vi "I(V)_K6221-K2182a_PK.vi"() -> ()   [LabVIEW 2016]
uses:
  Labview Drivers/Keithley 622x LV 2009/Keithley 622x.lvlib
panel:
  in  "Numeric Average":i32=50
  in  "wait (ms)":u32=1000
  out "Iset (A)":dbl=-4.3999999999999985e-06
  out "Vmeas (V)":dbl=-1.0767123e-06
  in  "Folder":path=path "D:/Banabir/Second round/14-04-2021"
  in  "Set Compliance voltage (V)":dbl=2.0 min=0.0 step=0.1 format="%_3f"
  out "I vs V":cluster{dbl, "Field Reading":dbl}[](graph)=[{-2.65213861e-07, "Field Reading"=0.0}, {-2.06331562e-07, "Field Reading"=1e-07}, {-2.45753416e-07, "Field Reading"=2e-07}, {-2.41658661e-07, "Field Reading"=3e-07}, {-2.45242211e-07, "Field Reading"=4e-07}, {-2.44727893e-07, "Field Reading"=5e-07}, {-1.955806e-07, "Field Reading"=6e-07}, {-2.17089385e-07, "Field Reading"=7e-07}, {-2.81598074e-07, "Field Reading"=8e-07}, {-2.74937155e-07, "Field Reading"=9e-07}, {-2.57527922e-07, "Field Reading"=1e-06}, {-1.97112335e-07, "Field Reading"=1.1e-06}, {-1.8175889e-07, "Field Reading"=1.2e-06}, {-2.14527365e-07, "Field Reading"=1.2999999999999998e-06}, {-1.61276589e-07, "Field Reading"=1.3999999999999997e-06}, {-5.88852258e-08, "Field Reading"=1.4999999999999996e-06}, {4.14620688e-08, "Field Reading"=1.5999999999999995e-06}, {4.55608442e-08, "Field Reading"=1.6999999999999994e-06}, {1.10074806e-07, "Field Reading"=1.7999999999999993e-06}, {9.16432587e-08, "Field Reading"=1.8999999999999992e-06}, {2.22710882e-07, "Field Reading"=1.999999999999999e-06}, {2.90806804e-07, "Field Reading"=2.099999999999999e-06}, {2.74933923e-07, "Field Reading"=2.199999999999999e-06}, {2.81079697e-07, "Field Reading"=2.2999999999999987e-06}, {3.16914884e-07, "Field Reading"=2.3999999999999986e-06}, {2.95409204e-07, "Field Reading"=2.4999999999999985e-06}, {3.58898183e-07, "Field Reading"=2.5999999999999984e-06}, {3.56848457e-07, "Field Reading"=2.6999999999999983e-06}, {4.40815949e-07, "Field Reading"=2.799999999999998e-06}, {4.45430022e-07, "Field Reading"=2.899999999999998e-06}, {4.50042171e-07, "Field Reading"=2.999999999999998e-06}, {5.23763566e-07, "Field Reading"=3.099999999999998e-06}, {5.54477469e-07, "Field Reading"=3.1999999999999977e-06}, {5.89806137e-07, "Field Reading"=3.2999999999999976e-06}, {6.03627656e-07, "Field Reading"=3.3999999999999975e-06}, {6.54317135e-07, "Field Reading"=3.4999999999999974e-06}, {7.12174301e-07, "Field Reading"=3.5999999999999973e-06}, {7.36747564e-07, "Field Reading"=3.699999999999997e-06}, {8.03819501e-07, "Field Reading"=3.799999999999997e-06}, {8.68836656e-07, "Field Reading"=3.899999999999997e-06}, {9.59970204e-07, "Field Reading"=3.999999999999997e-06}, {9.96323249e-07, "Field Reading"=4.099999999999997e-06}, {1.07823925e-06, "Field Reading"=4.199999999999997e-06}, {1.11458965e-06, "Field Reading"=4.299999999999997e-06}, {1.11817613e-06, "Field Reading"=4.399999999999997e-06}, {1.23695717e-06, "Field Reading"=4.499999999999997e-06}, {1.24360737e-06, "Field Reading"=4.599999999999997e-06}, {1.27996158e-06, "Field Reading"=4.6999999999999965e-06}, {1.30914358e-06, "Field Reading"=4.799999999999996e-06}, {1.29941092e-06, "Field Reading"=4.899999999999996e-06}, {1.45659309e-06, "Field Reading"=4.999999999999996e-06}, {1.47759059e-06, "Field Reading"=5.099999999999996e-06}, {1.56462638e-06, "Field Reading"=5.199999999999996e-06}, {1.56923247e-06, "Field Reading"=5.299999999999996e-06}, {1.5958572e-06, "Field Reading"=5.399999999999996e-06}, {1.62196573e-06, "Field Reading"=5.499999999999996e-06}, {1.65985372e-06, "Field Reading"=5.5999999999999955e-06}, {1.66548618e-06, "Field Reading"=5.699999999999995e-06}, {1.73869841e-06, "Field Reading"=5.799999999999995e-06}, {1.75918207e-06, "Field Reading"=5.899999999999995e-06}, {1.82420779e-06, "Field Reading"=5.999999999999995e-06}, {1.87539735e-06, "Field Reading"=6.099999999999995e-06}, {2.02541342e-06, "Field Reading"=6.199999999999995e-06}, {2.05920615e-06, "Field Reading"=6.299999999999995e-06}, {2.0607414e-06, "Field Reading"=6.399999999999995e-06}, {2.09299708e-06, "Field Reading"=6.4999999999999945e-06}, {2.14470835e-06, "Field Reading"=6.599999999999994e-06}, {2.22560209e-06, "Field Reading"=6.699999999999994e-06}, {2.29164603e-06, "Field Reading"=6.799999999999994e-06}, {2.29522927e-06, "Field Reading"=6.899999999999994e-06}, {2.34898799e-06, "Field Reading"=6.999999999999994e-06}, {2.35974308e-06, "Field Reading"=7.099999999999994e-06}, {2.33516555e-06, "Field Reading"=7.199999999999994e-06}, {2.38277613e-06, "Field Reading"=7.299999999999994e-06}, {2.52971809e-06, "Field Reading"=7.3999999999999935e-06}, {2.52562488e-06, "Field Reading"=7.499999999999993e-06}, {2.53073687e-06, "Field Reading"=7.599999999999993e-06}, {2.67562896e-06, "Field Reading"=7.699999999999994e-06}, {2.75038341e-06, "Field Reading"=7.799999999999995e-06}, {2.77444721e-06, "Field Reading"=7.899999999999996e-06}, {2.86045666e-06, "Field Reading"=7.999999999999996e-06}, {2.95312204e-06, "Field Reading"=8.099999999999997e-06}, {2.99612267e-06, "Field Reading"=8.199999999999998e-06}, {2.98793425e-06, "Field Reading"=8.299999999999998e-06}, {3.08214364e-06, "Field Reading"=8.4e-06}, {3.07036496e-06, "Field Reading"=8.5e-06}, {3.17481336e-06, "Field Reading"=8.6e-06}, {3.13692748e-06, "Field Reading"=8.700000000000001e-06}, {3.13795104e-06, "Field Reading"=8.800000000000002e-06}, {3.21679593e-06, "Field Reading"=8.900000000000003e-06}, {3.24444364e-06, "Field Reading"=9.000000000000004e-06}, {3.34223395e-06, "Field Reading"=9.100000000000004e-06}, {3.37244308e-06, "Field Reading"=9.200000000000005e-06}, {3.49890549e-06, "Field Reading"=9.300000000000006e-06}, {3.5705844e-06, "Field Reading"=9.400000000000007e-06}, {3.56136e-06, "Field Reading"=9.500000000000007e-06}, {3.64941777e-06, "Field Reading"=9.600000000000008e-06}, {3.65403077e-06, "Field Reading"=9.700000000000009e-06}, {3.70881304e-06, "Field Reading"=9.80000000000001e-06}, {3.74413912e-06, "Field Reading"=9.90000000000001e-06}, {3.78202672e-06, "Field Reading"=1.0000000000000011e-05}, {3.77588359e-06, "Field Reading"=1.0100000000000012e-05}, {3.79482737e-06, "Field Reading"=1.0200000000000012e-05}, {3.84807257e-06, "Field Reading"=1.0300000000000013e-05}, {3.96326851e-06, "Field Reading"=1.0400000000000014e-05}, {4.02675375e-06, "Field Reading"=1.0500000000000015e-05}, {4.01548692e-06, "Field Reading"=1.0600000000000015e-05}, {4.03188336e-06, "Field Reading"=1.0700000000000016e-05}, {4.11892625e-06, "Field Reading"=1.0800000000000017e-05}, {4.16499723e-06, "Field Reading"=1.0900000000000018e-05}, {4.13786622e-06, "Field Reading"=1.1000000000000018e-05}, {4.15936464e-06, "Field Reading"=1.1100000000000019e-05}, {4.15372248e-06, "Field Reading"=1.120000000000002e-05}, {4.1921208e-06, "Field Reading"=1.130000000000002e-05}, {4.20441259e-06, "Field Reading"=1.1400000000000021e-05}, {4.22285166e-06, "Field Reading"=1.1500000000000022e-05}, {4.41023425e-06, "Field Reading"=1.1600000000000023e-05}, {4.43121181e-06, "Field Reading"=1.1700000000000024e-05}, {4.48548487e-06, "Field Reading"=1.1800000000000024e-05}, {4.51827063e-06, "Field Reading"=1.1900000000000025e-05}, {4.56332253e-06, "Field Reading"=1.2000000000000026e-05}, {4.56996768e-06, "Field Reading"=1.2100000000000026e-05}, {4.61196138e-06, "Field Reading"=1.2200000000000027e-05}, {4.66060156e-06, "Field Reading"=1.2300000000000028e-05}, {4.71282017e-06, "Field Reading"=1.2400000000000029e-05}, {4.72562207e-06, "Field Reading"=1.250000000000003e-05}, {4.80549203e-06, "Field Reading"=1.260000000000003e-05}, {4.84132842e-06, "Field Reading"=1.2700000000000031e-05}, {4.81931379e-06, "Field Reading"=1.2800000000000032e-05}, {4.91812376e-06, "Field Reading"=1.2900000000000032e-05}, {4.97443564e-06, "Field Reading"=1.3000000000000033e-05}, {5.06864178e-06, "Field Reading"=1.3100000000000034e-05}, {5.15414621e-06, "Field Reading"=1.3200000000000035e-05}, {5.14594912e-06, "Field Reading"=1.3300000000000035e-05}, {5.15516684e-06, "Field Reading"=1.3400000000000036e-05}, {5.24221524e-06, "Field Reading"=1.3500000000000037e-05}, {5.29853469e-06, "Field Reading"=1.3600000000000038e-05}, {5.35638168e-06, "Field Reading"=1.3700000000000038e-05}, {5.37020179e-06, "Field Reading"=1.3800000000000039e-05}, {5.3492118e-06, "Field Reading"=1.390000000000004e-05}, {5.39375972e-06, "Field Reading"=1.400000000000004e-05}, {5.47056068e-06, "Field Reading"=1.4100000000000041e-05}, {5.50895206e-06, "Field Reading"=1.4200000000000042e-05}, {5.5514459e-06, "Field Reading"=1.4300000000000043e-05}, {5.55707986e-06, "Field Reading"=1.4400000000000043e-05}, {5.60366331e-06, "Field Reading"=1.4500000000000044e-05}, {5.64206701e-06, "Field Reading"=1.4600000000000045e-05}, {5.75061982e-06, "Field Reading"=1.4700000000000046e-05}, {5.78440485e-06, "Field Reading"=1.4800000000000046e-05}, {5.84225116e-06, "Field Reading"=1.4900000000000047e-05}, {5.85863506e-06, "Field Reading"=1.5000000000000048e-05}, {5.91290279e-06, "Field Reading"=1.5100000000000049e-05}, {5.90009794e-06, "Field Reading"=1.520000000000005e-05}, {5.99225908e-06, "Field Reading"=1.530000000000005e-05}, {6.0357811e-06, "Field Reading"=1.540000000000005e-05}, {6.09005686e-06, "Field Reading"=1.5500000000000048e-05}, {6.16276569e-06, "Field Reading"=1.5600000000000047e-05}, {6.223172e-06, "Field Reading"=1.5700000000000046e-05}, {6.27077906e-06, "Field Reading"=1.5800000000000045e-05}, {6.31429835e-06, "Field Reading"=1.5900000000000044e-05}, {6.34911719e-06, "Field Reading"=1.6000000000000043e-05}, {6.38342782e-06, "Field Reading"=1.6100000000000042e-05}, {6.40851838e-06, "Field Reading"=1.620000000000004e-05}, {6.46738862e-06, "Field Reading"=1.630000000000004e-05}, {6.49911838e-06, "Field Reading"=1.640000000000004e-05}, {6.55799613e-06, "Field Reading"=1.650000000000004e-05}, {6.62046237e-06, "Field Reading"=1.6600000000000038e-05}, {6.63786331e-06, "Field Reading"=1.6700000000000037e-05}, {6.73360462e-06, "Field Reading"=1.6800000000000036e-05}, {6.76740248e-06, "Field Reading"=1.6900000000000035e-05}, {6.79761286e-06, "Field Reading"=1.7000000000000034e-05}, {6.87696878e-06, "Field Reading"=1.7100000000000033e-05}, {6.92663472e-06, "Field Reading"=1.7200000000000032e-05}, {6.96504415e-06, "Field Reading"=1.730000000000003e-05}, {7.05310834e-06, "Field Reading"=1.740000000000003e-05}, {7.1360323e-06, "Field Reading"=1.750000000000003e-05}, {7.18210114e-06, "Field Reading"=1.7600000000000028e-05}, {7.20208147e-06, "Field Reading"=1.7700000000000027e-05}, {7.28861423e-06, "Field Reading"=1.7800000000000026e-05}, {7.33519871e-06, "Field Reading"=1.7900000000000025e-05}, {7.44937016e-06, "Field Reading"=1.8000000000000024e-05}, {7.48215567e-06, "Field Reading"=1.8100000000000023e-05}, {7.55229248e-06, "Field Reading"=1.8200000000000022e-05}, {7.5732755e-06, "Field Reading"=1.830000000000002e-05}, {7.68847322e-06, "Field Reading"=1.840000000000002e-05}, {7.65775525e-06, "Field Reading"=1.850000000000002e-05}, {7.67208615e-06, "Field Reading"=1.860000000000002e-05}, {7.7637263e-06, "Field Reading"=1.8700000000000017e-05}, {7.84923772e-06, "Field Reading"=1.8800000000000017e-05}, {7.85384559e-06, "Field Reading"=1.8900000000000016e-05}, {7.90913653e-06, "Field Reading"=1.9000000000000015e-05}, {7.93422015e-06, "Field Reading"=1.9100000000000014e-05}, {8.02791857e-06, "Field Reading"=1.9200000000000013e-05}, {8.06375894e-06, "Field Reading"=1.9300000000000012e-05}, {8.08936091e-06, "Field Reading"=1.940000000000001e-05}, {8.13646665e-06, "Field Reading"=1.950000000000001e-05}, {8.17230556e-06, "Field Reading"=1.960000000000001e-05}, {8.25165814e-06, "Field Reading"=1.9700000000000008e-05}, {8.28083444e-06, "Field Reading"=1.9800000000000007e-05}, {8.32742883e-06, "Field Reading"=1.9900000000000006e-05}, {8.40371126e-06, "Field Reading"=2e-05}, {8.32588703e-06, "Field Reading"=1.9900000000000003e-05}, {8.27059152e-06, "Field Reading"=1.9800000000000004e-05}, {8.24550498e-06, "Field Reading"=1.9700000000000005e-05}, {8.18766651e-06, "Field Reading"=1.9600000000000005e-05}, {8.16002117e-06, "Field Reading"=1.9500000000000006e-05}, {8.11034423e-06, "Field Reading"=1.9400000000000007e-05}, {8.06631431e-06, "Field Reading"=1.930000000000001e-05}, {7.96853626e-06, "Field Reading"=1.920000000000001e-05}, {7.96494837e-06, "Field Reading"=1.910000000000001e-05}, {7.88456389e-06, "Field Reading"=1.900000000000001e-05}, {7.84667228e-06, "Field Reading"=1.8900000000000012e-05}, {7.76577688e-06, "Field Reading"=1.8800000000000013e-05}, {7.72174608e-06, "Field Reading"=1.8700000000000014e-05}, {7.70996248e-06, "Field Reading"=1.8600000000000015e-05}, {7.64032909e-06, "Field Reading"=1.8500000000000016e-05}, {7.58196852e-06, "Field Reading"=1.8400000000000017e-05}, {7.52616124e-06, "Field Reading"=1.8300000000000018e-05}, {7.43451656e-06, "Field Reading"=1.820000000000002e-05}, {7.419165e-06, "Field Reading"=1.810000000000002e-05}, {7.41302153e-06, "Field Reading"=1.800000000000002e-05}, {7.40278217e-06, "Field Reading"=1.7900000000000022e-05}, {7.34748378e-06, "Field Reading"=1.7800000000000023e-05}, {7.26146266e-06, "Field Reading"=1.7700000000000024e-05}, {7.22614421e-06, "Field Reading"=1.7600000000000025e-05}, {7.15294258e-06, "Field Reading"=1.7500000000000026e-05}, {7.13912167e-06, "Field Reading"=1.7400000000000027e-05}, {7.05105581e-06, "Field Reading"=1.7300000000000027e-05}, {7.06896784e-06, "Field Reading"=1.720000000000003e-05}, {6.98551895e-06, "Field Reading"=1.710000000000003e-05}, {6.92254427e-06, "Field Reading"=1.700000000000003e-05}, {6.86724585e-06, "Field Reading"=1.690000000000003e-05}, {6.85240011e-06, "Field Reading"=1.6800000000000032e-05}, {6.78225464e-06, "Field Reading"=1.6700000000000033e-05}, {6.77713724e-06, "Field Reading"=1.6600000000000034e-05}, {6.69368315e-06, "Field Reading"=1.6500000000000035e-05}, {6.63224313e-06, "Field Reading"=1.6400000000000036e-05}, {6.64145914e-06, "Field Reading"=1.6300000000000037e-05}, {6.55391401e-06, "Field Reading"=1.6200000000000038e-05}, {6.54776972e-06, "Field Reading"=1.610000000000004e-05}, {6.44434302e-06, "Field Reading"=1.600000000000004e-05}, {6.37830276e-06, "Field Reading"=1.590000000000004e-05}, {6.32249712e-06, "Field Reading"=1.5800000000000042e-05}, {6.30507964e-06, "Field Reading"=1.5700000000000043e-05}, {6.27589889e-06, "Field Reading"=1.5600000000000044e-05}, {6.19193872e-06, "Field Reading"=1.5500000000000045e-05}, {6.14893632e-06, "Field Reading"=1.5400000000000046e-05}, {6.10695312e-06, "Field Reading"=1.5300000000000047e-05}, {6.07315478e-06, "Field Reading"=1.5200000000000046e-05}, {6.01376066e-06, "Field Reading"=1.5100000000000045e-05}, {6.01273927e-06, "Field Reading"=1.5000000000000044e-05}, {5.94362298e-06, "Field Reading"=1.4900000000000044e-05}, {5.89037156e-06, "Field Reading"=1.4800000000000043e-05}, {5.87757219e-06, "Field Reading"=1.4700000000000042e-05}, {5.83406487e-06, "Field Reading"=1.4600000000000041e-05}, {5.7818526e-06, "Field Reading"=1.450000000000004e-05}, {5.79054303e-06, "Field Reading"=1.440000000000004e-05}, {5.72397236e-06, "Field Reading"=1.430000000000004e-05}, {5.69632955e-06, "Field Reading"=1.4200000000000039e-05}, {5.62875043e-06, "Field Reading"=1.4100000000000038e-05}, {5.61902647e-06, "Field Reading"=1.4000000000000037e-05}, {5.53097021e-06, "Field Reading"=1.3900000000000036e-05}, {5.58626586e-06, "Field Reading"=1.3800000000000036e-05}, {5.5396681e-06, "Field Reading"=1.3700000000000035e-05}, {5.49102684e-06, "Field Reading"=1.3600000000000034e-05}, {5.46030697e-06, "Field Reading"=1.3500000000000033e-05}, {5.39784099e-06, "Field Reading"=1.3400000000000033e-05}, {5.28981952e-06, "Field Reading"=1.3300000000000032e-05}, {5.3456268e-06, "Field Reading"=1.3200000000000031e-05}, {5.23811359e-06, "Field Reading"=1.310000000000003e-05}, {5.28317073e-06, "Field Reading"=1.300000000000003e-05}, {5.23554661e-06, "Field Reading"=1.2900000000000029e-05}, {5.18742312e-06, "Field Reading"=1.2800000000000028e-05}, {5.16080263e-06, "Field Reading"=1.2700000000000027e-05}, {5.08911473e-06, "Field Reading"=1.2600000000000027e-05}, {5.02306725e-06, "Field Reading"=1.2500000000000026e-05}, {4.95087495e-06, "Field Reading"=1.2400000000000025e-05}, {4.89097002e-06, "Field Reading"=1.2300000000000025e-05}, {4.85103666e-06, "Field Reading"=1.2200000000000024e-05}, {4.81161312e-06, "Field Reading"=1.2100000000000023e-05}, {4.8223712e-06, "Field Reading"=1.2000000000000022e-05}, {4.71997748e-06, "Field Reading"=1.1900000000000022e-05}, {4.70513009e-06, "Field Reading"=1.1800000000000021e-05}, {4.61860758e-06, "Field Reading"=1.170000000000002e-05}, {4.50494221e-06, "Field Reading"=1.160000000000002e-05}, {4.50442328e-06, "Field Reading"=1.1500000000000019e-05}, {4.48907395e-06, "Field Reading"=1.1400000000000018e-05}, {4.48549552e-06, "Field Reading"=1.1300000000000017e-05}, {4.43275985e-06, "Field Reading"=1.1200000000000016e-05}, {4.37336829e-06, "Field Reading"=1.1100000000000016e-05}, {4.35544798e-06, "Field Reading"=1.1000000000000015e-05}, {4.23615778e-06, "Field Reading"=1.0900000000000014e-05}, {4.18496019e-06, "Field Reading"=1.0800000000000013e-05}, {4.13529928e-06, "Field Reading"=1.0700000000000013e-05}, {4.0963864e-06, "Field Reading"=1.0600000000000012e-05}, {4.10252432e-06, "Field Reading"=1.0500000000000011e-05}, {4.14245452e-06, "Field Reading"=1.040000000000001e-05}, {4.0723185e-06, "Field Reading"=1.030000000000001e-05}, {3.99655577e-06, "Field Reading"=1.0200000000000009e-05}, {3.91820595e-06, "Field Reading"=1.0100000000000008e-05}, {3.90693848e-06, "Field Reading"=1.0000000000000008e-05}, {3.90182893e-06, "Field Reading"=9.900000000000007e-06}, {3.89824771e-06, "Field Reading"=9.800000000000006e-06}, {3.89568225e-06, "Field Reading"=9.700000000000005e-06}, {3.82297919e-06, "Field Reading"=9.600000000000005e-06}, {3.79072008e-06, "Field Reading"=9.500000000000004e-06}, {3.75283128e-06, "Field Reading"=9.400000000000003e-06}, {3.74925146e-06, "Field Reading"=9.300000000000002e-06}, {3.69600662e-06, "Field Reading"=9.200000000000002e-06}, {3.68985764e-06, "Field Reading"=9.100000000000001e-06}, {3.53830951e-06, "Field Reading"=9e-06}, {3.48967903e-06, "Field Reading"=8.9e-06}, {3.4169754e-06, "Field Reading"=8.799999999999999e-06}, {3.35195893e-06, "Field Reading"=8.699999999999998e-06}, {3.26798993e-06, "Field Reading"=8.599999999999997e-06}, {3.32840376e-06, "Field Reading"=8.499999999999997e-06}, {3.28130617e-06, "Field Reading"=8.399999999999996e-06}, {3.22038204e-06, "Field Reading"=8.299999999999995e-06}, {3.19170899e-06, "Field Reading"=8.199999999999994e-06}, {3.14817946e-06, "Field Reading"=8.099999999999994e-06}, {3.06473437e-06, "Field Reading"=7.999999999999993e-06}, {3.0155901e-06, "Field Reading"=7.899999999999992e-06}, {2.89219787e-06, "Field Reading"=7.799999999999991e-06}, {2.84355222e-06, "Field Reading"=7.69999999999999e-06}, {2.79798017e-06, "Field Reading"=7.599999999999991e-06}, {2.73245105e-06, "Field Reading"=7.499999999999991e-06}, {2.68023355e-06, "Field Reading"=7.399999999999991e-06}, {2.76420187e-06, "Field Reading"=7.299999999999991e-06}, {2.74935814e-06, "Field Reading"=7.199999999999991e-06}, {2.68791939e-06, "Field Reading"=7.099999999999991e-06}, {2.63261821e-06, "Field Reading"=6.9999999999999914e-06}, {2.60291933e-06, "Field Reading"=6.8999999999999915e-06}, {2.51843848e-06, "Field Reading"=6.799999999999992e-06}, {2.5061508e-06, "Field Reading"=6.699999999999992e-06}, {2.33208474e-06, "Field Reading"=6.599999999999992e-06}, {2.3167298e-06, "Field Reading"=6.499999999999992e-06}, {2.30443977e-06, "Field Reading"=6.399999999999992e-06}, {2.24402212e-06, "Field Reading"=6.299999999999992e-06}, {2.26142112e-06, "Field Reading"=6.199999999999992e-06}, {2.24708744e-06, "Field Reading"=6.099999999999992e-06}, {2.18258492e-06, "Field Reading"=5.9999999999999925e-06}, {2.06226311e-06, "Field Reading"=5.899999999999993e-06}, {1.97317707e-06, "Field Reading"=5.799999999999993e-06}, {1.89791536e-06, "Field Reading"=5.699999999999993e-06}, {1.8943317e-06, "Field Reading"=5.599999999999993e-06}, {1.91123261e-06, "Field Reading"=5.499999999999993e-06}, {1.79142144e-06, "Field Reading"=5.399999999999993e-06}, {1.82674468e-06, "Field Reading"=5.299999999999993e-06}, {1.75353415e-06, "Field Reading"=5.199999999999993e-06}, {1.65932968e-06, "Field Reading"=5.0999999999999935e-06}, {1.65933232e-06, "Field Reading"=4.999999999999994e-06}, {1.54669792e-06, "Field Reading"=4.899999999999994e-06}, {1.44584143e-06, "Field Reading"=4.799999999999994e-06}, {1.52673386e-06, "Field Reading"=4.699999999999994e-06}, {1.4320141e-06, "Field Reading"=4.599999999999994e-06}, {1.40795279e-06, "Field Reading"=4.499999999999994e-06}, {1.32296227e-06, "Field Reading"=4.399999999999994e-06}, {1.08181445e-06, "Field Reading"=4.299999999999994e-06}, {1.07105849e-06, "Field Reading"=4.1999999999999945e-06}, {1.07361536e-06, "Field Reading"=4.099999999999995e-06}, {1.06030613e-06, "Field Reading"=3.999999999999995e-06}, {9.90675451e-07, "Field Reading"=3.899999999999995e-06}, {9.98353274e-07, "Field Reading"=3.799999999999995e-06}, {9.51769766e-07, "Field Reading"=3.699999999999995e-06}, {9.19007087e-07, "Field Reading"=3.599999999999995e-06}, {8.96477356e-07, "Field Reading"=3.4999999999999953e-06}, {8.37598555e-07, "Field Reading"=3.3999999999999954e-06}, {7.43906148e-07, "Field Reading"=3.2999999999999955e-06}, {7.07042824e-07, "Field Reading"=3.1999999999999956e-06}, {7.8384287e-07, "Field Reading"=3.0999999999999957e-06}, {6.97316697e-07, "Field Reading"=2.999999999999996e-06}, {6.99871857e-07, "Field Reading"=2.899999999999996e-06}, {6.61988855e-07, "Field Reading"=2.799999999999996e-06}, {6.67112949e-07, "Field Reading"=2.699999999999996e-06}, {5.21710306e-07, "Field Reading"=2.5999999999999963e-06}, {5.11980802e-07, "Field Reading"=2.4999999999999964e-06}, {5.26306067e-07, "Field Reading"=2.3999999999999965e-06}, {5.57538796e-07, "Field Reading"=2.2999999999999966e-06}, {5.49862592e-07, "Field Reading"=2.1999999999999967e-06}, {4.38246539e-07, "Field Reading"=2.099999999999997e-06}, {4.53099149e-07, "Field Reading"=1.999999999999997e-06}, {3.79374306e-07, "Field Reading"=1.899999999999997e-06}, {3.25102595e-07, "Field Reading"=1.7999999999999972e-06}, {2.04792301e-07, "Field Reading"=1.6999999999999973e-06}, {2.36019239e-07, "Field Reading"=1.5999999999999974e-06}, {2.33452923e-07, "Field Reading"=1.4999999999999975e-06}, {2.2372704e-07, "Field Reading"=1.3999999999999976e-06}, {2.67761542e-07, "Field Reading"=1.2999999999999977e-06}, {2.54450874e-07, "Field Reading"=1.1999999999999978e-06}, {1.63316468e-07, "Field Reading"=1.099999999999998e-06}, {7.72994096e-08, "Field Reading"=9.99999999999998e-07}, {8.85529671e-08, "Field Reading"=8.999999999999981e-07}, {7.06354729e-08, "Field Reading"=7.999999999999981e-07}, {1.87884609e-07, "Field Reading"=6.999999999999981e-07}, {1.58696118e-07, "Field Reading"=5.999999999999981e-07}, {1.73034013e-07, "Field Reading"=4.999999999999981e-07}, {1.02383086e-07, "Field Reading"=3.999999999999981e-07}, {6.60310964e-08, "Field Reading"=2.999999999999981e-07}, {1.43341752e-07, "Field Reading"=1.9999999999999809e-07}, {2.34987166e-07, "Field Reading"=9.999999999999809e-08}, {1.56651714e-07, "Field Reading"=-1.9058241313221758e-21}, {1.5204492e-07, "Field Reading"=-1.000000000000019e-07}, {2.03758966e-07, "Field Reading"=-2.000000000000019e-07}, {2.2474776e-07, "Field Reading"=-3.000000000000019e-07}, {1.65354644e-07, "Field Reading"=-4.000000000000019e-07}, {1.18764208e-07, "Field Reading"=-5.000000000000019e-07}, {7.88302354e-08, "Field Reading"=-6.000000000000019e-07}, {1.93518827e-07, "Field Reading"=-7.000000000000019e-07}, {1.5665572e-07, "Field Reading"=-8.000000000000019e-07}, {2.47273023e-07, "Field Reading"=-9.000000000000019e-07}, {2.08356789e-07, "Field Reading"=-1.0000000000000019e-06}, {2.10917939e-07, "Field Reading"=-1.1000000000000018e-06}, {1.69965974e-07, "Field Reading"=-1.2000000000000016e-06}, {1.11596254e-07, "Field Reading"=-1.3000000000000015e-06}, {9.20117195e-09, "Field Reading"=-1.4000000000000014e-06}, {-7.42491073e-08, "Field Reading"=-1.5000000000000013e-06}, {-7.5273293e-08, "Field Reading"=-1.6000000000000012e-06}, {-6.65732606e-08, "Field Reading"=-1.700000000000001e-06}, {-1.58906482e-08, "Field Reading"=-1.800000000000001e-06}, {-1.34670081e-07, "Field Reading"=-1.9000000000000009e-06}, {-2.32454805e-07, "Field Reading"=-2.0000000000000008e-06}, {-2.82111171e-07, "Field Reading"=-2.1000000000000006e-06}, {-3.47645977e-07, "Field Reading"=-2.2000000000000005e-06}, {-3.37922223e-07, "Field Reading"=-2.3000000000000004e-06}, {-3.85029026e-07, "Field Reading"=-2.4000000000000003e-06}, {-2.86727063e-07, "Field Reading"=-2.5e-06}, {-2.61119956e-07, "Field Reading"=-2.6e-06}, {-2.56507099e-07, "Field Reading"=-2.7e-06}, {-3.87066578e-07, "Field Reading"=-2.8e-06}, {-5.12512258e-07, "Field Reading"=-2.8999999999999998e-06}, {-5.18652063e-07, "Field Reading"=-2.9999999999999997e-06}, {-5.77529798e-07, "Field Reading"=-3.0999999999999995e-06}, {-6.54844775e-07, "Field Reading"=-3.1999999999999994e-06}, {-6.1951305e-07, "Field Reading"=-3.2999999999999993e-06}, {-6.40503708e-07, "Field Reading"=-3.399999999999999e-06}, {-6.31290379e-07, "Field Reading"=-3.499999999999999e-06}, {-6.56374953e-07, "Field Reading"=-3.599999999999999e-06}, {-6.85558188e-07, "Field Reading"=-3.699999999999999e-06}, {-7.71570974e-07, "Field Reading"=-3.7999999999999988e-06}, {-9.11853044e-07, "Field Reading"=-3.899999999999999e-06}, {-9.0314763e-07, "Field Reading"=-3.999999999999999e-06}, {-9.40523971e-07, "Field Reading"=-4.099999999999999e-06}, {-1.02704958e-06, "Field Reading"=-4.199999999999999e-06}, {-1.0767123e-06, "Field Reading"=-4.299999999999999e-06}]
  out "data":dbl[](array[numeric])=[-1.0767123e-06, -4.299999999999999e-06, 0.25039820930232565]
  in  "Nanovoltmeter 2182a VISA":refnum<visa-resource-name>="COM1"
  in  "Current source K6221 VISA":refnum<visa-resource-name>="COM1"
  in  "Step":dbl[](array[numeric])=[1e-07, 1e-07, 1e-07, 1e-07, 1e-07] min=-3000.0 max=3000.0 format="%.1e"
  in  "To":dbl[](array[numeric])=[2e-05, -2e-05, 2e-05, -2e-05, 0.0] min=-3000.0 max=3000.0 format="%.1e"
  in  "From":dbl[](array[numeric])=[0.0, 2e-05, -2e-05, 2e-05, -2e-05] min=-3000.0 max=3000.0 format="%.1e"
  in  "file name":string="013_NTJJ03_DC_IV_350mK_I_2-3_V_9-8"
  out "File path":path=path "D:/Banabir/Second round/14-04-2021/013_NTJJ03_DC_IV_350mK_I_2-3_V_9-8.dat"
  # ".dat"
  # "Set Current (A)"
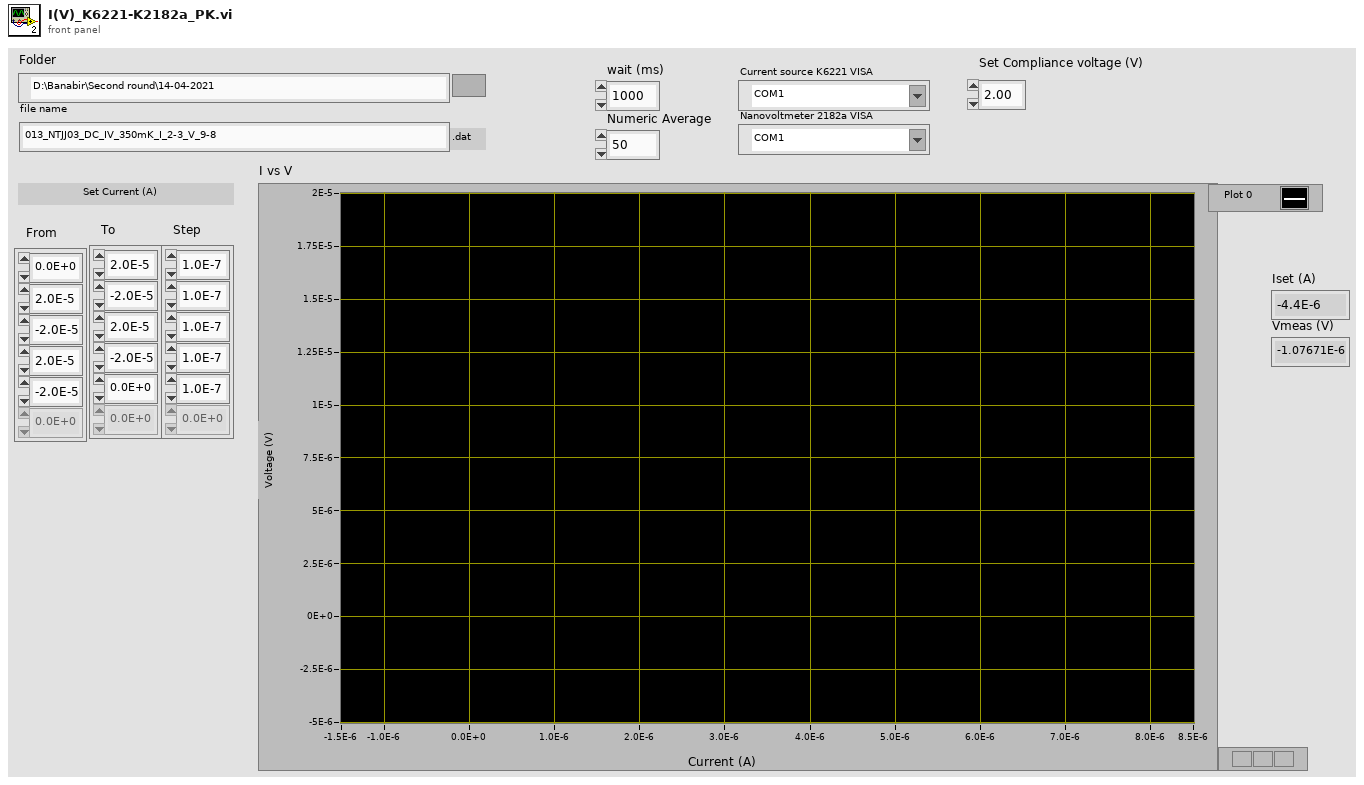
[diagram p1: front panel]
types:
  T1 = enum16{"open", "replace", "create", "open or create", "replace or create", "replace or create with confirmation"}
  T2 = typedef "Keithley 622x.lvlib/KE622x -- Current Level.ctl" = dbl
  T3 = cluster{"Average value":dbl, "Average value":dbl}
  T4 = cluster{"Average value":dbl, "Average value":dbl}[]
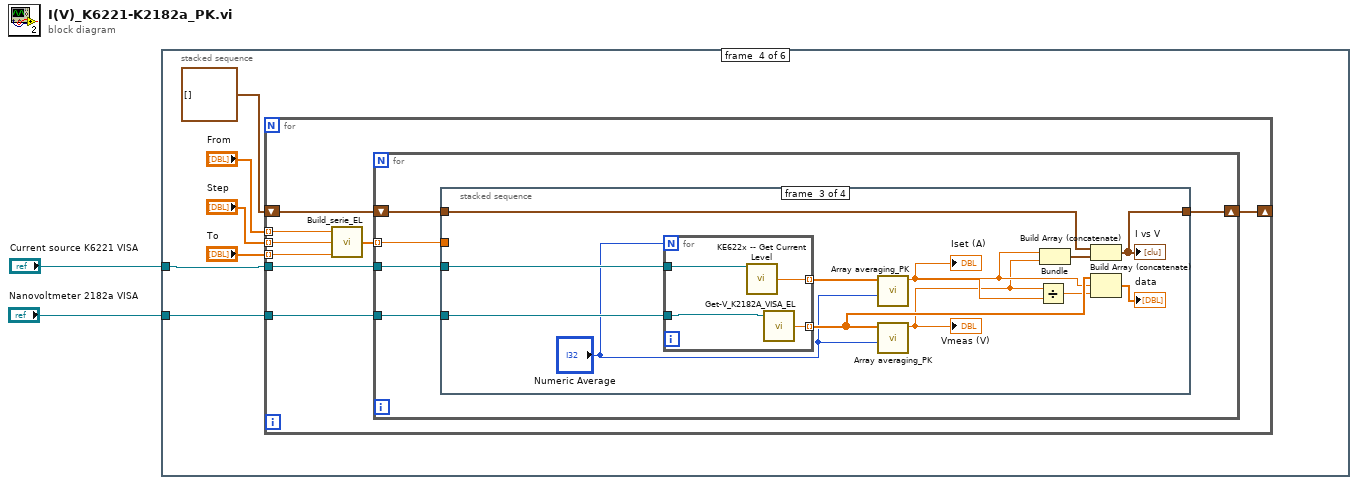
[diagram p0: block diagram]
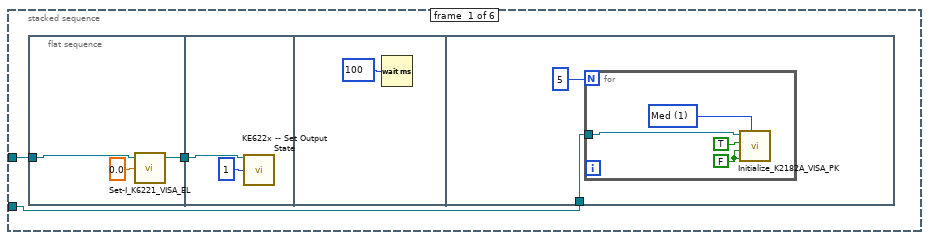
[diagram p2: hidden frame]
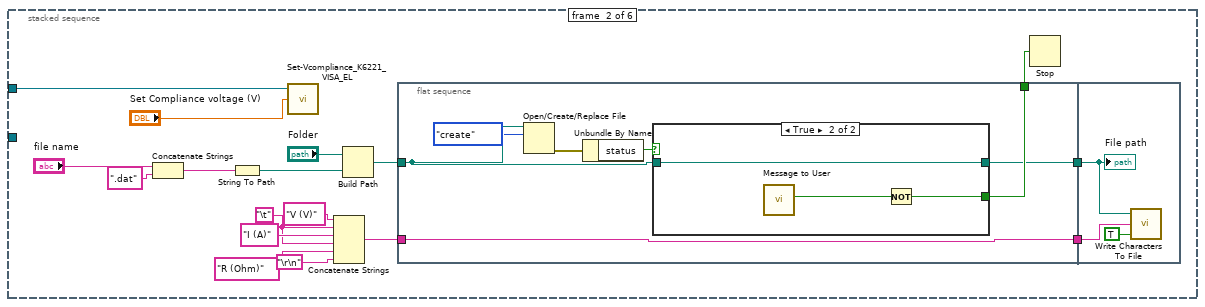
[diagram p3: hidden frame]
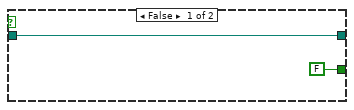
[diagram p4: hidden frame]
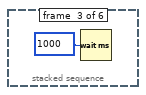
[diagram p5: hidden frame]
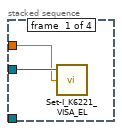
[diagram p6: hidden frame]
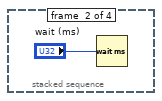
[diagram p7: hidden frame]
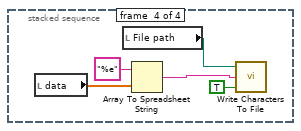
[diagram p8: hidden frame]
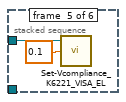
[diagram p9: hidden frame]
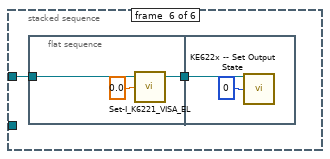
[diagram p10: hidden frame]
diagram:
  n1 = stacked-sequence {
    tunnel: "Nanovoltmeter 2182a VISA" -> [w3 _ _ w53 _ _]
    tunnel: "Current source K6221 VISA" -> [w4 w24 _ w52 w95 w97]
    frame #0 {
      n2 = flat-sequence {
        tunnel: w4 -> [w8]
        tunnel: [w6] -> w5
        tunnel: w5 -> [w10]
        tunnel: w3 -> [w12]
        frame #0 {
          n3 = call "Set-I_K6221_VISA_EL.vi"("Set I (A)"=0.0, "K6221 VISA"=w8) -> ("K6221 VISA out"=w6:refnum<visa-resource-name>)  [unwired: 2 in, 1 out]
        }
        frame #1 {
          n4 = call "KE622x -- Set Output State.vi"("Resource In"=w10, "Output State"=1) -> ()  [unwired: 12 in, 2 out]
        }
        frame #2 {
          n5 = Wait (ms)(milliseconds to wait=100) -> ()  [unwired: 1 out]
        }
        frame #3 {
          n6 = for {
            N: 5 ("Numeric") -> [_]
            tunnel: w12 -> [w14]
            w16 = u16 1 items=["Slow", "Med", "Fast"] ("Rate (NPLC)")
            w17 = FALSE ("Auto range?")
            n7 = call "Initialize_K2182A_VISA_PK.vi"("VISA address"=w14, "Auto range?"=TRUE, "Analog LPass\nFilter?"=w17, "DC\nFilter?"=w17, "Rate (NPLC)"=w16) -> ()  [unwired: 2 in]
          }
        }
      }
    }
    frame #1 {
      w25 = "\t"
      n8 = Concatenate Strings("file name", ".dat" ("string")) -> (w31:string)
      n9 = String To Path(string=w31) -> (path=w19:path)
      n10 = call "Set-Vcompliance_K6221_VISA_EL.vi"("Set Compliance voltage (V)"="Set Compliance voltage (V)", "K6221 VISA"=w24) -> ()  [unwired: 2 in, 2 out]
      n11 = Concatenate Strings("V (V)" ("string"), w25, "I (A)" ("string"), w25, "R (Ohm)" ("string"), "\r\n") -> (w32:string)
      n12 = Build Path(base path="Folder", name or relative path=w19) -> (appended path=w18:path)
      n13 = flat-sequence {
        tunnel: w18 -> [w38]
        tunnel: w32 -> [w41]
        tunnel: [w41] -> w34
        tunnel: [w40] -> w29
        tunnel: [w39] -> w33
        tunnel: w34 -> [w48]
        tunnel: w33 -> [w47]
        frame #0 {
          n14 = Open/Create/Replace File(file path (use dialog)=w38, operation (0:open)=T1."create") -> (error out=w37:errorcluster)  [unwired: 4 in, 2 out]
          n15 = Unbundle By Name(w37) -> ("status"=w35:bool)
          n16 = case shown="True" w35 {
            tunnel: [FALSE ("Yes") w45] -> w40
            tunnel: [w42 w44] -> w39
            tunnel: w38 -> [w42 w44]
            frame False {
            }
            frame True {
              n17 = call "Message to User"() -> ("Yes"=w46:bool)  [unwired: 10 in, 1 out]
              n18 = Not(x=w46) -> (.not. x?=w45:bool)
            }
          }
        }
        frame #1 {
          n19 = call <vilib>:"Write Characters To File.vi"("append to file? (new file:F)"=TRUE, "character string"=w48, "file path (dialog if empty)"=w47) -> ()  [unwired: 2 in, 1 out]
          "File path" <- w47
        }
      }
      n20 = Stop(stop? (T)=w29) -> ()
    }
    frame #2 {
      n21 = Wait (ms)(milliseconds to wait=u32 1000) -> ()  [unwired: 1 out]
    }
    frame #3 {
      n22 = for {
        tunnel: "From" -> [w59] mode=indexing
        tunnel: "To" -> [w58] mode=indexing
        tunnel: "Step" -> [w57] mode=indexing
        tunnel: w53 -> [w64]
        tunnel: w52 -> [w63]
        shift-right: [w61] -> _
        shift-left: cluster{dbl, "Field Reading":dbl}[] [] -> [w62]
        n23 = call "Build_serie_EL.vi"("end value"=w58, "increment"=w57, "start value"=w59) -> ("output array"=w60:dbl[])
        n24 = for {
          tunnel: w60 -> [w67] mode=indexing
          tunnel: w64 -> [w69]
          tunnel: w63 -> [w68]
          shift-right: [w65] -> w61
          shift-left: w62 -> [w66]
          n25 = stacked-sequence {
            tunnel: w69 -> [_ _ w79 _]
            tunnel: w68 -> [w71 _ w78 _]
            tunnel: w66 -> [_ _ w82 _]
            tunnel: w67 -> [w70 _ _ _]
            tunnel: [_ _ w81 _] -> w65
            frame #0 {
              n26 = call "Set-I_K6221_VISA_EL.vi"("Set I (A)"=w70, "K6221 VISA"=w71) -> ()  [unwired: 2 in, 2 out]
            }
            frame #1 {
              n27 = Wait (ms)(milliseconds to wait="wait (ms)") -> ()  [unwired: 1 out]
            }
            frame #2 {
              n28 = for {
                N: "Numeric Average" -> [_]
                tunnel: [w88] -> w80 mode=indexing
                tunnel: w79 -> [w87]
                tunnel: w78 -> [w86]
                tunnel: [w85] -> w77 mode=indexing
                n29 = call "KE622x -- Get Current Level.vi"("Resource In"=w86) -> ("Current Level (A)"=w85:T2)  [unwired: 12 in, 2 out]
                n30 = call "Get-V_K2182A_VISA_EL.vi"("VISA K2182A"=w87) -> ("V (V)"=w88:dbl)  [unwired: 2 in, 2 out]
              }
              n31 = call "Array averaging_PK.vi"("Number averaging"="Numeric Average", "numeric array"=w77) -> ("Average value"=w74:dbl)  [unwired: 9 in]
              "Iset (A)" <- w74
              n32 = call "Array averaging_PK.vi"("Number averaging"="Numeric Average", "numeric array"=w80) -> ("Average value"=w73:dbl)  [unwired: 9 in]
              "Vmeas (V)" <- w73
              n33 = Divide(x=w73, y=w74) -> (x/y=w75:dbl)
              n34 = Bundle("Average value"=w74, "Average value"=w73) -> (w83:T3)  [unwired: 1 in]
              n35 = Build Array (concatenate)(w82, w83) -> (w81:T4)
              "I vs V" <- w81
              n36 = Build Array (concatenate)(w80, w74, w75) -> (→"data":dbl[])
            }
            frame #3 {
              n37 = local read "data"() -> (w89:dbl[])
              n38 = local read "File path"() -> (w91:path)
              n39 = Array To Spreadsheet String(array=w89, 3:"%e" ("format string")) -> (spreadsheet string=w92:string)  [unwired: 1 in]
              n40 = call <vilib>:"Write Characters To File.vi"("append to file? (new file:F)"=TRUE, "character string"=w92, "file path (dialog if empty)"=w91) -> ()  [unwired: 2 in, 1 out]
            }
          }
        }
      }
    }
    frame #4 {
      n41 = call "Set-Vcompliance_K6221_VISA_EL.vi"("Set Compliance voltage (V)"=0.1, "K6221 VISA"=w95) -> ()  [unwired: 2 in, 2 out]
    }
    frame #5 {
      n42 = flat-sequence {
        tunnel: w97 -> [w100]
        tunnel: [w98] -> w96
        tunnel: w96 -> [w102]
        frame #0 {
          n43 = call "Set-I_K6221_VISA_EL.vi"("Set I (A)"=0.0, "K6221 VISA"=w100) -> ("K6221 VISA out"=w98:refnum<visa-resource-name>)  [unwired: 2 in, 1 out]
        }
        frame #1 {
          n44 = call "KE622x -- Set Output State.vi"("Resource In"=w102, "Output State"=0) -> ()  [unwired: 12 in, 2 out]
        }
      }
    }
  }
